vi "programa3.vi"() -> ()   [LabVIEW 2011]
panel:
  out "Observacion":string
  in  "Numeric":dbl
  out "Boolean":bool
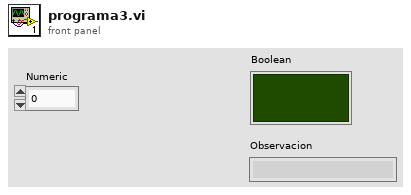
[diagram p1: front panel]
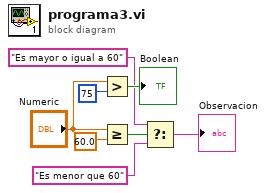
[diagram p0: block diagram]
diagram:
  n1 = Greater?(x="Numeric", y=75) -> (0:→"Boolean":bool)
  n2 = Greater Or Equal?(x="Numeric", y=60.0) -> (x >= y?=w4:bool)
  n3 = Select(t="Es mayor o igual a 60", s=w4, f="Es menor que 60") -> (s? t:f=→"Observacion":string)
